vi "CMWtestsubscribeBOOL.vi"(8 "error in (no error)":errorcluster, 11 "URL":string="VAC.VGHA_41677/PR") -> (0 "error out":errorcluster)   [LabVIEW 2014]
uses:
  <userlib>/_RADE/RIO/CMW/classes/CMWSubscribe/openCMWSubscribe.vi
  <userlib>/_RADE/RIO/CMW/classes/CMWSubscribe/CMWSubscribe.vi
  <userlib>/_RADE/RIO/CMW/classes/CMWSubscribe/CMWSubscribe.lvclass
panel:
  out "length":i32
  out "Boolean":bool
  out "Data":variant
  out "Loop":i32
  in  "stop":bool
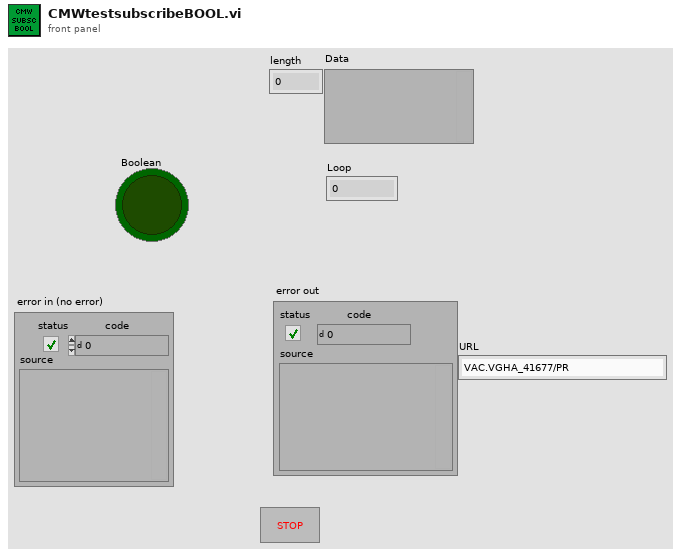
[diagram p1: front panel]
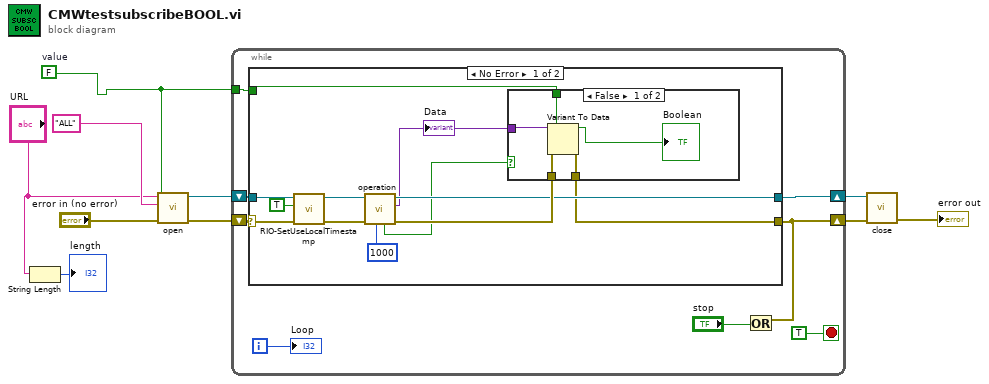
[diagram p0: block diagram]
diagram:
  w3 = FALSE  # value
  n1 = String Length(string="URL") -> (length=→"length":i32)
  n2 = call-poly <userlib>:"open.vi"("error in (no error)"="error in (no error)", "Data type"=w3, "Cycle"="ALL", "URL"="URL") -> ("error out"=w8:errorcluster, "Object out"=w7:refnum<class "CMWSubscribe.lvclass">)  [unwired: 6 in]
  n3 = while {
    shift-right: [w16] -> w6
    shift-left: w8 -> [w18]
    shift-right: [w14] -> w5
    shift-left: w7 -> [w15]
    tunnel: w3 -> [w13]
    i -> [w17]
    stop <- TRUE stop-if-true
    n4 = case shown="No Error" w18 {
      selector: w18 -> [w23 w38]
      tunnel: [w28 w38] -> w16
      tunnel: w15 -> [w21 w37]
      tunnel: [w29 w37] -> w14
      tunnel: w13 -> [w27 _]
      frame No Error {
        n5 = call-dynamic "RIO-SetUseLocalTimestamp.vi"("error in (no error)"=w23, "Use Local Timestamp?"=TRUE, "CMWBase in"=w21) -> ("error out"=w22:errorcluster, "CMWBase out"=w20:refnum<class "CMWSubscribe.lvclass">)  [unwired: 7 in]
        n6 = call-poly <userlib>:"operation.vi"("Timeout (10000 ms)"=1000, "error in (no error)"=w22, "Object in"=w20) -> ("error out"=w30:errorcluster, "Data"=w26:variant, "Object out"=w29:refnum<class "CMWSubscribe.lvclass">, "Timeout?"=w24:bool)  [unwired: 4 in, 1 out]
        "Data" <- w26
        n7 = case shown="False" w24 {
          tunnel: w30 -> [w35 w36]
          tunnel: [w34 w36] -> w28
          tunnel: w26 -> [w33 _]
          tunnel: w27 -> [w32 _]
          frame False {
            n8 = Variant To Data(error in=w35, type=w32, Variant=w33) -> (data=→"Boolean":bool, error out=w34:errorcluster)
          }
          frame True {
          }
        }
      }
      frame Error {
      }
    }
    n9 = Or(x=w16, y="stop") -> ()  [unwired: 1 out]
    "Loop" <- w17
  }
  n10 = call-dynamic "close.vi"("error in (no error)"=w6, "Object in"=w5) -> ("error out"=→"error out":errorcluster)  [unwired: 9 in]
